vi "Example - Method API.vi"() -> ()   [LabVIEW 2011]
uses:
  Taskbar Progress Bar.xctl
panel:
  in  "Progress Bar":bool
  in  "Taskbar Progress Bar":u64(xcontrol)
  in  "Progress Bar Maximum":u64=100
  # "Taskbar Progress  XControl"
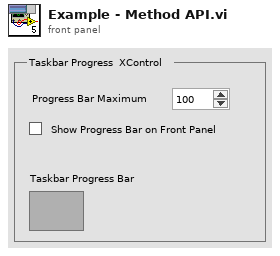
[diagram p1: front panel]
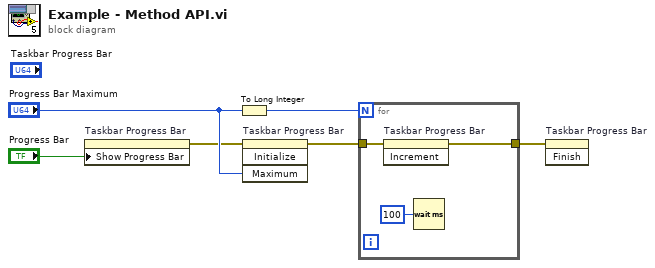
[diagram p0: block diagram]
diagram:
  n1 = property on="Taskbar Progress Bar" class="Taskbar Progress Bar (strict)"("Show Progress Bar"="Progress Bar") -> (error out=w2:errorcluster)  [unwired: 2 in, 1 out]
  n2 = To Long Integer(number="Progress Bar Maximum") -> (32bit integer=w5:i32)
  n3 = invoke on="Taskbar Progress Bar" class="Taskbar Progress Bar (strict)" method="Initialize"(error in=w2, "Maximum"="Progress Bar Maximum") -> (error out=w3:errorcluster)  [unwired: 2 in, 3 out]
  n4 = for {
    N: w5 -> [_]
    tunnel: w3 -> [w8]
    tunnel: [w7] -> w1
    n5 = invoke on="Taskbar Progress Bar" class="Taskbar Progress Bar (strict)" method="Increment"(error in=w8) -> (error out=w7:errorcluster)  [unwired: 2 in, 2 out]
    n6 = Wait (ms)(milliseconds to wait=u32 100) -> ()  [unwired: 1 out]
  }
  n7 = invoke on="Taskbar Progress Bar" class="Taskbar Progress Bar (strict)" method="Finish"(error in=w1) -> ()  [unwired: 2 in, 3 out]
